vi "SOUR_POW_ALC_MODE.vi"(0 "VISA IN":refnum<visa-resource-name>, 1 "Port number":i32, 2 "ALC Mode":string, 3 "Source Port":string, 5 "error in":errorcluster, 7 "Channel":i32) -> (14 "VISA Out":refnum<visa-resource-name>, 19 "error out":errorcluster)   [LabVIEW 2018, in "PNA-X.lvlib"]
doc: "SOURce<cnum>:POWer<port>:ALC[:MODE] <char>, [src] \n1824\n\n(Read-Write) Sets and returns the ALC mode for the specified channel and port. Use \nSOUR:POW:ALC:MODE:CAT? to return a list of valid ALC modes for the PNA. \nLearn more about ALC mode. \nParameters \n<cnum> Any existing channel number. If unspecified, value is set to 1 \n<port> Port number of the PNA. If unspecified, value is set to 1. To make settings for \nports that are not simple numbers, use the [src] argument. \n<char> ALC Mode. \nFor the PNA-X choose from: \nINTernal Standard ALC loop \nOPENloop No ALC loop \n[src] String. (NOT case sensitive). Source port. Optional. Use SOUR:CAT? to \nreturn a list of valid port names. \nWhile this argument can be used to make settings for ALL ports, it is designed \nto access ports that are not simple numbers, such as \"Port 1 Src2\". Otherwise, \nthe <port> argument performs the same function. If both arguments are \nspecified, [src] takes priority. \nExamples SOUR:POW:ALC INT \nsource2:power2:alc:mode openloop \nsource:power:alc:mode openloop,\"Port 1 Src2\" \nQuery Syntax SOURce<cnum>:POWer<port>:ALC:MODE? [src] \nReturn Type Character \nDefault INTernal"
uses:
  PNA-X.lvlib
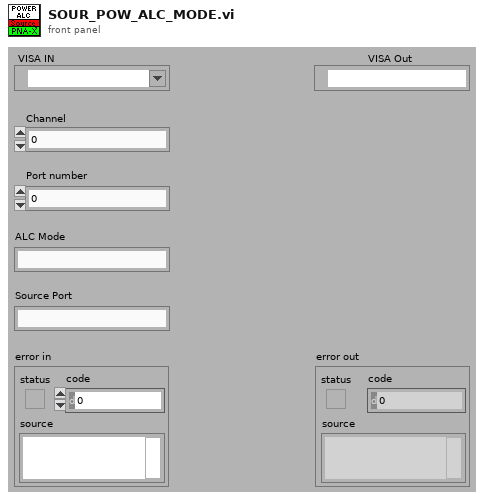
[diagram p1: front panel]
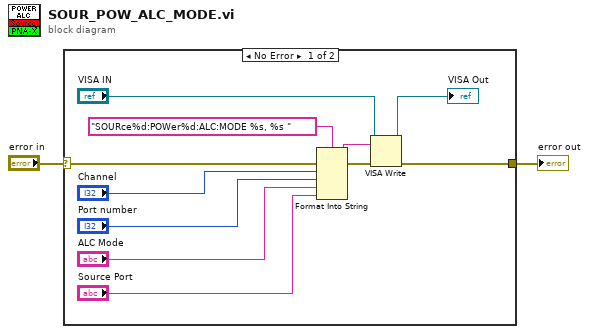
[diagram p0: block diagram]
diagram:
  n1 = case shown="No Error" "error in" {
    selector: "error in" -> [w13 w14]
    tunnel: [w8 w14] -> w1
    frame No Error {
      n2 = Format Into String(format string="SOURce%d:POWer%d:ALC:MODE %s, %s " ("Cmdline"), error in=w13, "Channel", "Port number", "ALC Mode", "Source Port") -> (resulting string=w11:string, error out=w12:errorcluster)  [unwired: 1 in]
      n3 = VISA Write(VISA resource name="VISA IN", write buffer=w11, error in (no error)=w12) -> (VISA resource name out=→"VISA Out":refnum<visa-resource-name>, error out=w8:errorcluster)  [unwired: 1 out]
    }
    frame Error {
    }
  }
  "error out" <- w1
